vi "Set pannel updating false.vi"(5 "error in":errorcluster, 6 "Index(0)":i32) -> (1 "error out":errorcluster)   [LabVIEW 2011]
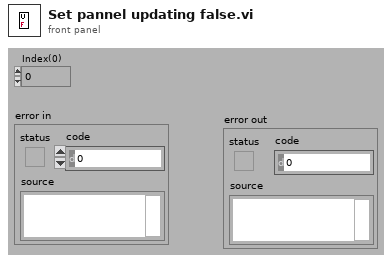
[diagram p1: front panel]
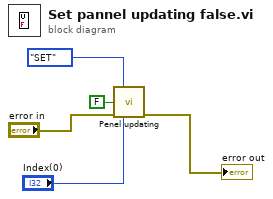
[diagram p0: block diagram]
diagram:
  n1 = call "Penel updating.vi"("Action(GET)"=enum16{"GET", "SET"}."SET", "Panel updating in"=FALSE, "error in (no error)"="error in", "Index(0)"="Index(0)") -> ("error out"=→"error out":errorcluster)  [unwired: 10 in, 1 out]
